vi "Log Errors and Warnings.vi"(8 "error in (no error)":errorcluster, 11 "Async Handler in":refnum<class "Async Handler.lvclass">) -> (0 "error out":errorcluster, 3 "Async Handler out":refnum<class "Async Handler.lvclass">)   [LabVIEW 2020, in "Async Handler.lvclass"]
uses:
  Async Handler.lvclass
  Logging/Logging.lvclass
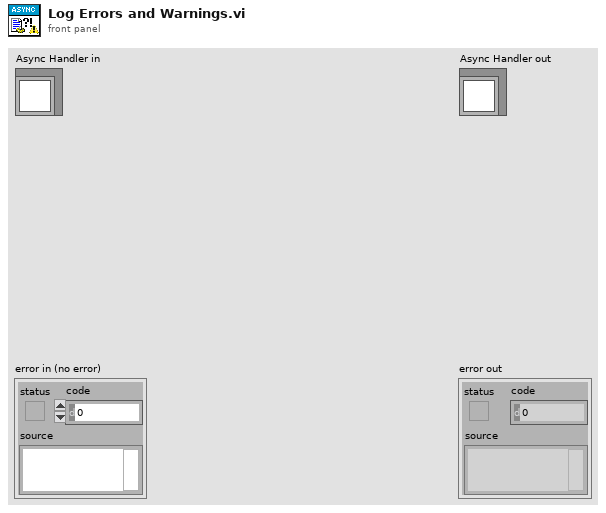
[diagram p1: front panel]
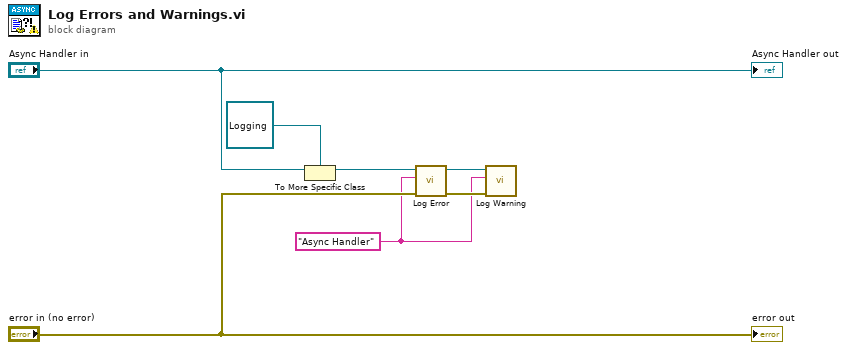
[diagram p0: block diagram]
diagram:
  w1 = "Async Handler" ("format string")
  n1 = To More Specific Class(target class=refnum<class "Logging.lvclass"> refnum ("Logging.lvclass"), reference="Async Handler in") -> (specific class reference=w5:refnum<class "Logging.lvclass">)  [unwired: 1 in, 1 out]
  n2 = call "Log Error.vi"("error in (no error)"="error in (no error)", "Message"=w1, "Logging In"=w5) -> ("error out"=w2:errorcluster, "Logging Out"=w3:refnum<class "Logging.lvclass">)  [unwired: 7 in]
  n3 = call "Log Warning.vi"("error in (no error)"=w2, "Message"=w1, "Logging In"=w3) -> ()  [unwired: 7 in, 2 out]
  "error out" <- "error in (no error)"
  "Async Handler out" <- "Async Handler in"
